vi "Calibration Parameter.vi"(8 "error in (no error)":errorcluster, 9 "Frequency (20)":dbl=20.0 min=20.0 max=1000000.0 format="%.2f", 11 "VISA resource name":refnum<visa-resource-name>) -> (0 "error out":errorcluster, 1 "Kc":dbl format="%^.2e", 3 "VISA resource name out":refnum<visa-resource-name>)   [LabVIEW 2015, in "Agilent 428X Series.lvlib"]
doc: "This VI computes the value of calibration interpolation factor Kc.\nIf current Frequency is equal to one of the preset direct calibration frequencies, the result will be 0. All other frequencies value will make Kc equal to 0.0003 \n\nDisclaimer: All accuracy calculation VI's are not part of the original \n driver. They are provided for supplementry purpose only.\n If user desires very high accuracy data, please do or \n check the calculation seperately."
uses:
  Agilent 428X Series.lvlib
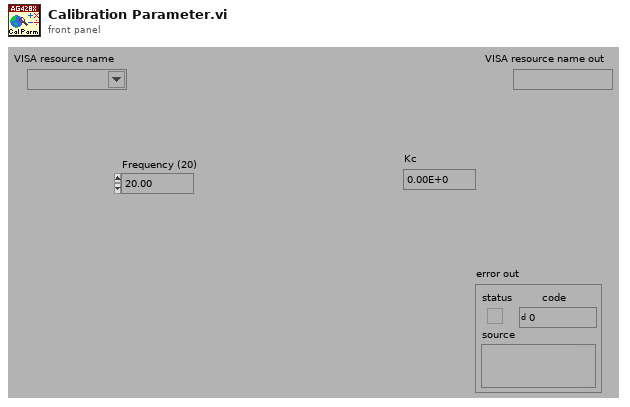
[diagram p1: front panel]
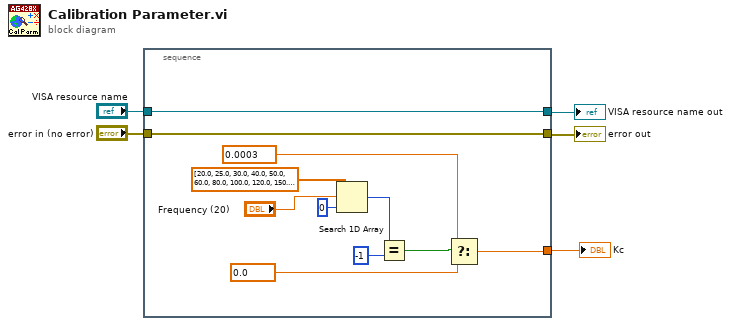
[diagram p0: block diagram]
diagram:
  n1 = stacked-sequence {
    tunnel: "error in (no error)" -> [w15]
    tunnel: "VISA resource name" -> [w16]
    tunnel: [w16] -> w3
    tunnel: [w15] -> w2
    tunnel: [w9] -> w1
    frame #0 {
      n2 = Search 1D Array(1D array=dbl[] [20.0, 25.0, 30.0, 40.0, 50.0, 60.0, 80.0, 100.0, 120.0, 150.0, 200.0, 250.0, 300.0, 400.0, 500.0, 600.0, 800.0, 1000.0, 1200.0, 1500.0, 2000.0, 2500.0, 3000.0, 4000.0, 5000.0, 6000.0, 8000.0, 10000.0, 12000.0, 15000.0, 20000.0, 25000.0, 30000.0, 40000.0, 50000.0, 60000.0, 80000.0, 100000.0, 120000.0, 150000.0, 200000.0, 250000.0, 300000.0, 400000.0, 500000.0, 600000.0, 800000.0, 1000000.0], element="Frequency (20)", start index (0)=0) -> (index of element=w12:i32)
      n3 = Equal?(x=w12, y=-1) -> (x = y?=w10:bool)
      n4 = Select(t=0.0003, s=w10, f=0.0) -> (s? t:f=w9:dbl)
    }
  }
  "error out" <- w2
  "VISA resource name out" <- w3
  "Kc" <- w1
